vi "Get All Nodes in a Generation.vi"(8 "error in":errorcluster, 10 "Generation":i32, 11 "XML Document in":refnum<class "XML Document.lvclass">) -> (0 "error out":errorcluster, 2 "Nodes":refnum<class "Node.lvclass">[](array[class]), 3 "XML Document out":refnum<class "XML Document.lvclass">)   [LabVIEW 2014, in "XML Document.lvclass"]
uses:
  XML Document.lvclass
  Node_class/Node.lvclass
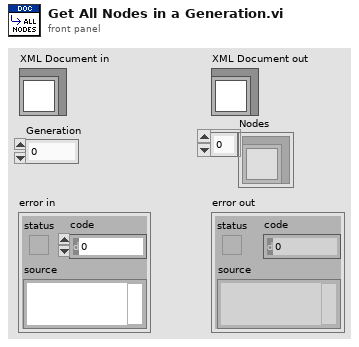
[diagram p1: front panel]
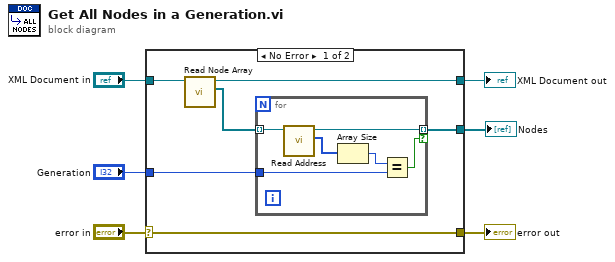
[diagram p0: block diagram]
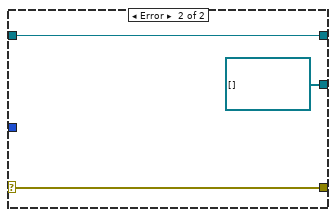
[diagram p2: hidden frame]
diagram:
  n1 = case shown="No Error" "error in" {
    selector: "error in" -> [w11 w21]
    tunnel: [w11 w21] -> w5
    tunnel: [w10 w20] -> w3
    tunnel: "XML Document in" -> [w12 w20]
    tunnel: "Generation" -> [w8 _]
    tunnel: [w7 refnum<class "Node.lvclass">[] []] -> w1
    frame No Error {
      n2 = call-dynamic "Read Node Array.vi"("XML Document in"=w12) -> ("Node Array"=w9:refnum<class "Node.lvclass">[], "XML Document out"=w10:refnum<class "XML Document.lvclass">)  [unwired: 8 in, 1 out]
      n3 = for {
        tunnel: w9 -> [w18] mode=indexing
        tunnel: w8 -> [w16]
        tunnel: [w13] -> w7 mode=indexing if=w14
        n4 = call-dynamic "Read Address.vi"("Node in"=w18) -> ("Address"=w15:i32[], "Node out"=w13:refnum<class "Node.lvclass">)  [unwired: 8 in, 1 out]
        n5 = Array Size(array=w15) -> (size(s)=w17:i32)
        n6 = Equal?(x=w17, y=w16) -> (x = y?=w14:bool)
      }
    }
    frame Error {
    }
  }
  "error out" <- w5
  "XML Document out" <- w3
  "Nodes" <- w1
